vi "WriteI2C.vi"(4 "Byte 3":u8, 6 "Byte 2":u8, 8 "error in (no error)":errorcluster, 9 "Pin":T1=2 items=["D2"=2, "D3"=3, "D4"=4, "D5"=5, "D6"=6, "D7"=7, "D8"=8, "D9"=9, "A0"=14, "A1"=15, "A2"=16, "A3"=17], 10 "Command":T2=1 items=["Digital Read"=1, "Digital Write"=2, "Analog Read"=3, "Analog Write"=4, "Pin Mode"=5, "Ultrasonic Read"=7, "Version"=8, "Dust Sensor Read"=10, "Encoder Read"=11, "Flow Read"=12, "Flow Disabled"=13, "Dust Sensor Enable"=14, "Dust Sensor Disable"=15, "Encoder Enable"=16, "Encoder Disable"=17, "Flow Enable"=18, "Accelerometer Read"=20, "RTC Read"=30, "DHT Read"=40], 11 "GrovePi in":refnum<class "GrovePi.lvclass">) -> (0 "error out":errorcluster, 2 "Message":u8[](array[numeric]) format="%.0x", 3 "GrovePi out":refnum<class "GrovePi.lvclass">)   [LabVIEW 2014, in "GrovePi.lvclass"]
doc: "Writes a command to the GrovePi over the I2C bus."
uses:
  GrovePi.lvclass
  Command.ctl
  Pin.ctl
  GrovePi.lvclass/GrovePi.ctl
  I2C/I2C.lvclass
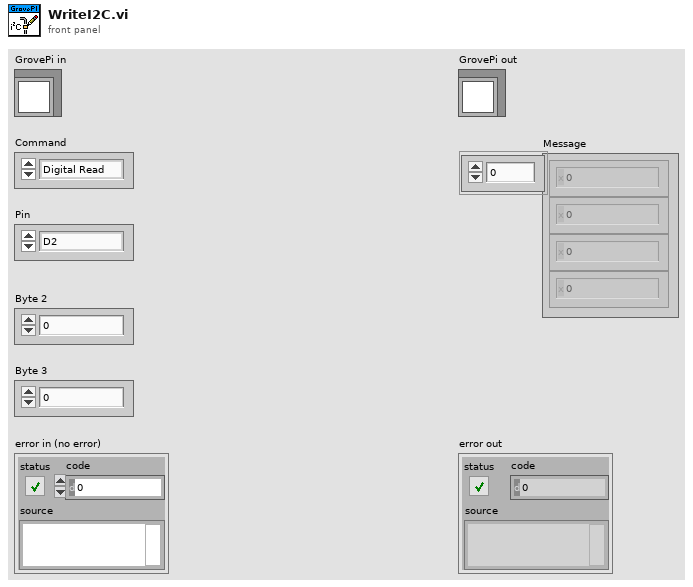
[diagram p1: front panel]
types:
  T1 = typedef "GrovePi.lvclass/Pin.ctl" = u8
  T2 = typedef "GrovePi.lvclass/Command.ctl" = u8
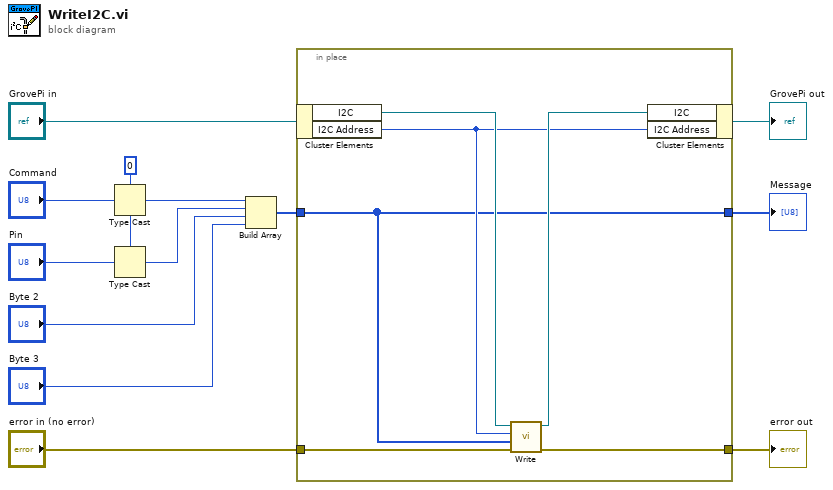
[diagram p0: block diagram]
diagram:
  w7 = u8 0 ("Byte 2")
  n1 = Type Cast(type=w7, x="Command") -> (*(type *) &x=w10:u8)
  n2 = Type Cast(type=w7, x="Pin") -> (*(type *) &x=w8:u8)
  n3 = Build Array(w10, w8, "Byte 2", "Byte 3") -> (w5:u8[])
  n4 = in-place {
    in-place-border: "error in (no error)" -> [w19]
    in-place-border: [w15] -> w1
    in-place-border: w5 -> [w14]
    in-place-border: [w14] -> w4
    n5 = in-place-cluster #1("GrovePi in") -> ("I2C"=w18:refnum<class "I2C.lvclass">, "I2C Address"=w16:u8)
    n6 = call-dynamic "Write.vi"("error in (no error)"=w19, "Data"=w14, "I2C Slave Address"=w16, "I2C in"=w18) -> ("error out"=w15:errorcluster, "I2C out"=w17:refnum<class "I2C.lvclass">)  [unwired: 6 in]
    n7 = in-place-cluster #1("I2C"=w17, "I2C Address"=w16) -> (→"GrovePi out":refnum<class "GrovePi.lvclass">)
  }
  "Message" <- w4
  "error out" <- w1
